vi "Set Axis Displacement Units.vi"(4 "Units (Encoder Count)":T1(ring), 5 "error in (no error)":errorcluster, 7 "Axis (1)":i32=1 min=1 max=3, 8 "VISA resource name":refnum<visa-resource-name>) -> (0 "error out":errorcluster, 3 "VISA resource name out":refnum<visa-resource-name>)   [LabVIEW 2018, in "Newport ESP301.lvlib"]
doc: "This command is used to set the displacement units for the for axis <B>Axis (1)</B>.\n<B>NOTE:</B>The unit of measure as used with this controller is intended as a label only. It is the user’s responsibility to convert and resend all affected parameters (e.g., velocity, acceleration, etc…) when switching from one unit of measure to another."
uses:
  Newport ESP301.lvlib
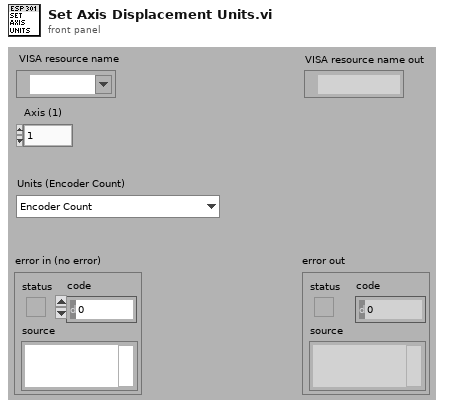
[diagram p1: front panel]
types:
  T1 = enum16{"Encoder Count", "Motor Step", "millimeter", "micrometer", "inch", "milli-inch", "micro-inch", "degree", "gradian", "radian", "milliradian", "microradian"}
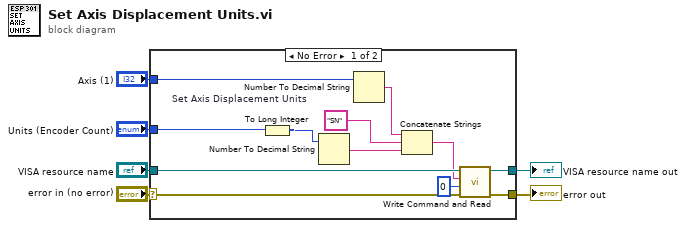
[diagram p0: block diagram]
diagram:
  n1 = case shown="No Error" "error in (no error)" {
    selector: "error in (no error)" -> [w17 w20]
    tunnel: [w16 w20] -> w5
    tunnel: "VISA resource name" -> [w18 w19]
    tunnel: [w15 w19] -> w3
    tunnel: "Axis (1)" -> [w11 _]
    tunnel: "Units (Encoder Count)" -> [w8 _]
    frame No Error {
      w13 = "SN"  # Set Axis Displacement Units
      n2 = To Long Integer(number=w8) -> (32bit integer=w7:i32)
      n3 = Number To Decimal String(number=w7) -> (decimal integer string=w14:string)  [unwired: 1 in]
      n4 = Number To Decimal String(number=w11) -> (decimal integer string=w12:string)  [unwired: 1 in]
      n5 = Concatenate Strings(w12, w13, w14) -> (w10:string)
      n6 = call "Write Command and Read.vi"("error in (no error)"=w17, "Bytes to read (100)"=u32 0, "Command"=w10, "VISA resource name"=w18) -> ("error out"=w16:errorcluster, "VISA resource name out"=w15:refnum<visa-resource-name>)  [unwired: 3 in, 1 out]
    }
    frame Error {
    }
  }
  "error out" <- w5
  "VISA resource name out" <- w3
